vi "AutoFeedForwardConversion.vi"(1 "Target Velocity (in/s)":dbl) -> (0 "Equivalent Joystick Command (ul)":dbl)   [LabVIEW 2020]
doc: "Converts the feed-forward path goal velocity from inches/sec to a unitless drive command. This VI is intended for use with the FRC 4265 Autonomous Path Planner and the pure-pursuit algorithm. The input is in inches per second and the output is a unitless equivalent joystick command."
uses:
  autoninfo.vi
  robotconstants.vi
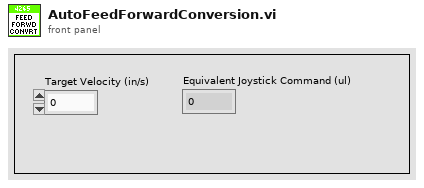
[diagram p1: front panel]
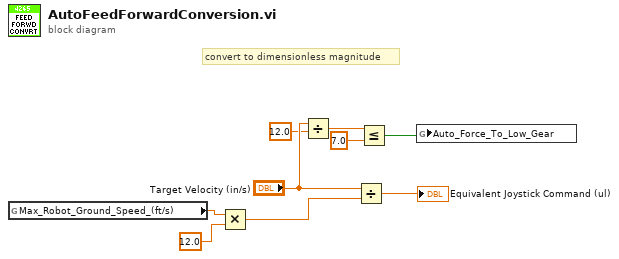
[diagram p0: block diagram]
diagram:
  # "convert to dimensionless magnitude"
  n1 = global read "robotconstants.vi" "Max_Robot_Ground_Speed_(ft/s)"() -> (w1:dbl)
  n2 = Multiply(x=w1, y=12.0) -> (x*y=w7:dbl)
  n3 = Divide(x="Target Velocity (in/s)", y=12.0) -> (x/y=w4:dbl)
  n4 = Divide(x="Target Velocity (in/s)", y=w7) -> (x/y=→"Equivalent Joystick Command (ul)":dbl)
  n5 = Less Or Equal?(x=w4, y=7.0) -> (x <= y?=w2:bool)
  n6 = global write "autoninfo.vi" "Auto_Force_To_Low_Gear"(w2) -> ()
